vi "Temperature controller top level_v3.vi"() -> ()   [LabVIEW 2015]
uses:
  heating or cooling.vi
  <vilib>/Utility/file.llb/Write Delimited Spreadsheet (DBL).vi
  Heating or cooling global.vi
  <vilib>/Utility/file.llb/Write Delimited Spreadsheet (string).vi
panel:
  in  "?":bool
  in  "Time step":u32=2000
  in  "Comments":string="DTLquad5_run1"
  in  "TSetpoint":sgl=50.0
  in  "file path (dialog if empty)":path=path "C:/Temperature cycling test data/DTLquad5_run2"
  in  "error in":errorcluster
  out "Tcurrent":dbl(slide)=37.65891647338867 scale=0.0..100.0
  out "Tambient":dbl(slide)=23.492000579833984 scale=0.0..100.0
  out "Tambient":sgl=23.492
  out "Tcurrent":sgl=37.658916
  out "error out":errorcluster {"code" format="%.0x"}
  out "Current iteration":i32
  in  "Number of iterations":i32=5
  in  "Current limit":dbl=10.6 caption="Current"
  in  "Voltage":dbl=15.0 format="%#_13g"
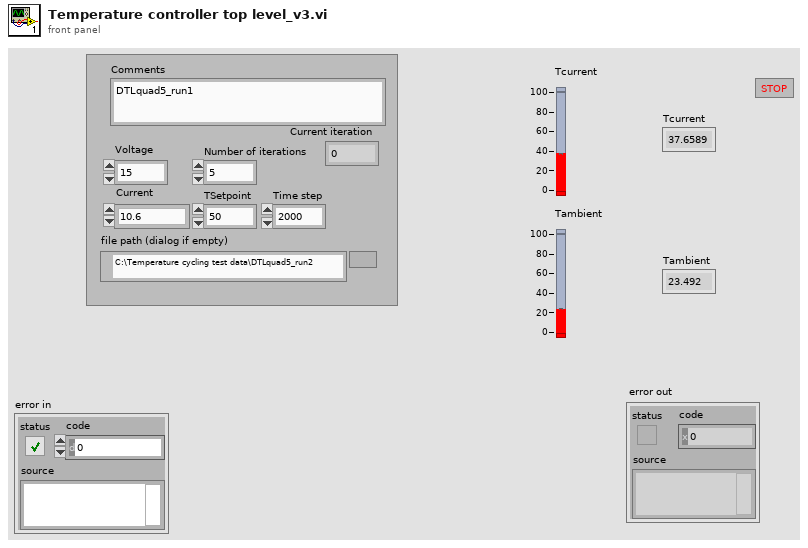
[diagram p1: front panel]
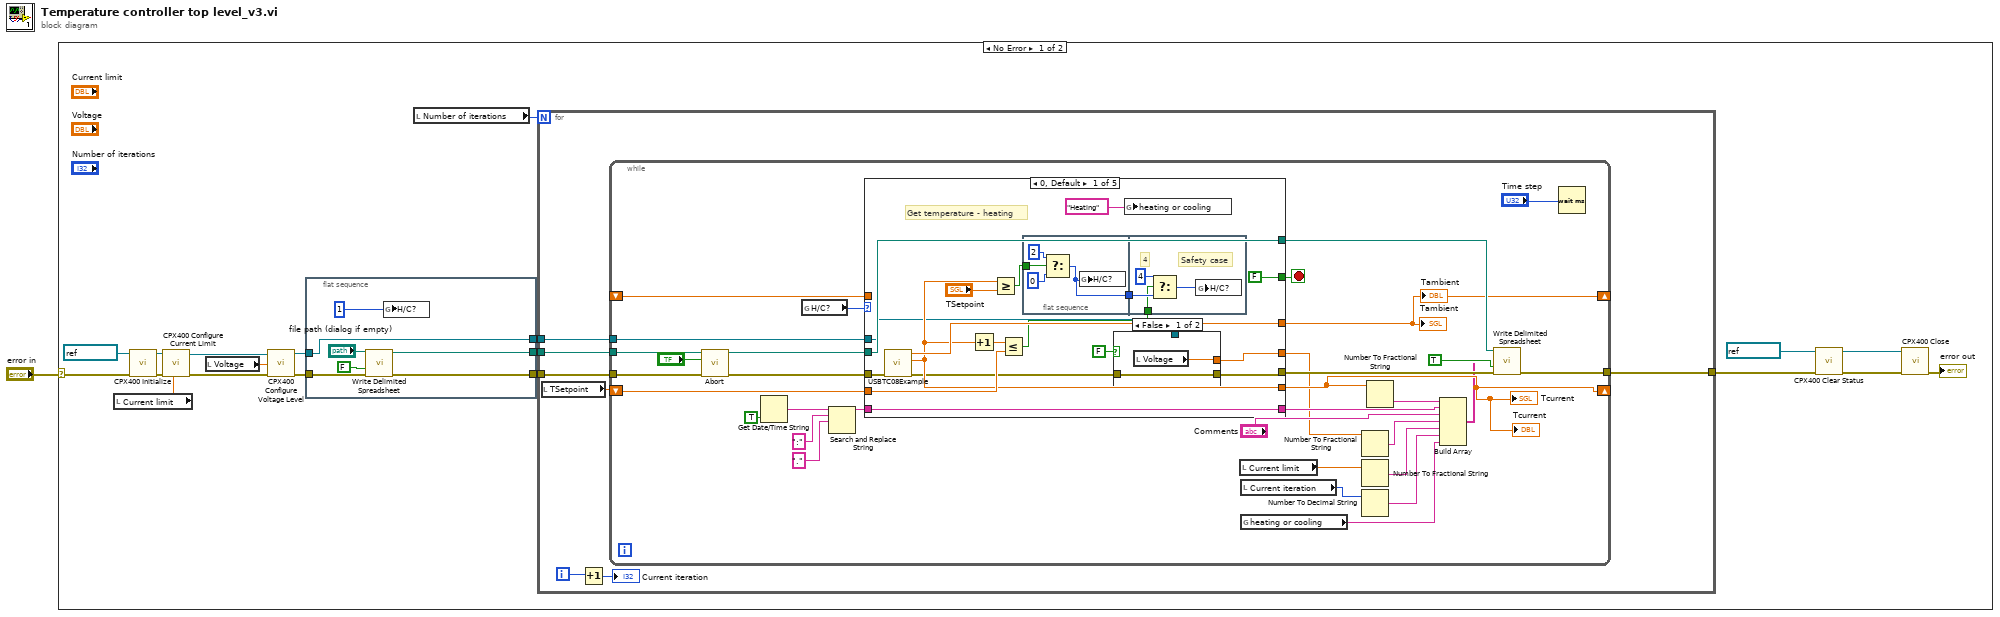
[diagram p0: block diagram]
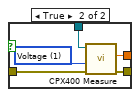
[diagram p2: hidden frame]
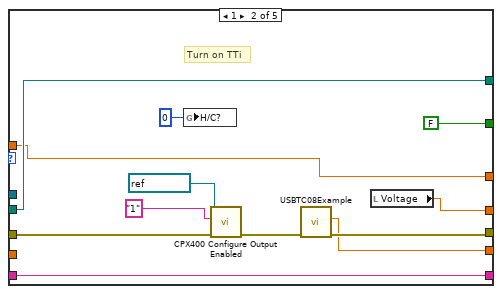
[diagram p3: hidden frame]
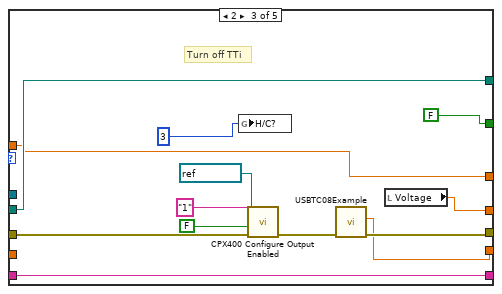
[diagram p4: hidden frame]
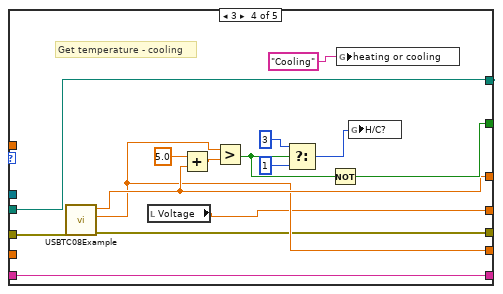
[diagram p5: hidden frame]
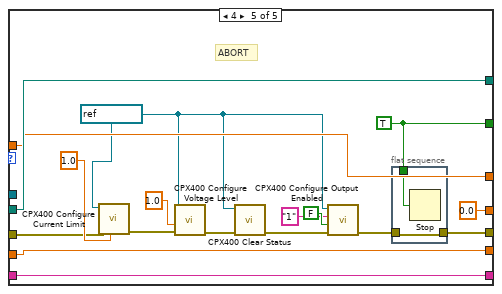
[diagram p6: hidden frame]
diagram:
  n1 = case shown="No Error" "error in" {
    selector: "error in" -> [w7 _]
    frame No Error {
      n2 = local read "Current limit"() -> (w16:dbl)
      n3 = call <instrlib>:"CPX400 Initialize.vi"("error in (no error)"=w7, "resource name"=refnum<k15> "COM5") -> ("error out"=w15:errorcluster, "instrument handle out"=w14:refnum<k15>)  [unwired: 8 in]
      n4 = call <instrlib>:"CPX400 Configure Current Limit.vi"("limit (1.0)"=w16, "error in (no error)"=w15, "instrument handle"=w14) -> ("error out"=w18:errorcluster, "instrument handle out"=w19:refnum<k15>)  [unwired: 7 in]
      n5 = local read "Voltage"() -> (w17:dbl)
      n6 = call <instrlib>:"CPX400 Configure Voltage Level.vi"("error in (no error)"=w18, "level (1.0)"=w17, "instrument handle"=w19) -> ("error out"=w10:errorcluster, "instrument handle out"=w12:refnum<k15>)  [unwired: 7 in]
      n7 = flat-sequence {
        tunnel: w12 -> [w21]
        tunnel: [w24] -> w11
        tunnel: w10 -> [w25]
        tunnel: [w23] -> w9
        tunnel: [w21] -> w6
        frame #0 {
          n8 = call-poly <vilib>:"Write Delimited Spreadsheet.vi"("file path (dialog if empty)"="file path (dialog if empty)", "append to file? (F)"=FALSE, "error in (no error)"=w25) -> ("new file path (Not A Path if cancelled)"=w23:path, "error out"=w24:errorcluster)  [unwired: 11 in]
          n9 = global write "heating or cooling.vi" "H/C?"(u8 1 ("heating or cooling")) -> ()
        }
      }
      n10 = local read "Number of iterations"() -> (w13:i32)
      n11 = for {
        N: w13 -> [_]
        tunnel: w11 -> [w34]
        tunnel: w9 -> [w33]
        tunnel: [w32] -> w5
        tunnel: w6 -> [w28]
        i -> [w30]
        n12 = local read "TSetpoint"() -> (w31:sgl)
        n13 = Increment(x=w30) -> (x+1=→"Current iteration":i32)
        n14 = while {
          tunnel: w34 -> [w37]
          shift-right: [w50] -> _
          shift-left: w31 -> [w65]
          tunnel: w33 -> [w57]
          tunnel: [w56] -> w32
          shift-right: [w53] -> _
          shift-left: _ -> [w54]
          tunnel: w28 -> [w38]
          stop <- w66 stop-if-true
          n15 = call "Abort.vi"("error in"=w37, "stop"="?") -> ("error in 2"=w36:errorcluster)  [unwired: 9 in]
          n16 = Get Date/Time String(want seconds? (F)=TRUE) -> (time string=w63:string)  [unwired: 2 in, 1 out]
          n17 = global read "heating or cooling.vi" "H/C?"() -> (w52:u8)
          n18 = Search and Replace String(input string=w63, search string=":", replace string="." ("replace string (\"\")")) -> (result string=w60:string)  [unwired: 5 in, 3 out]
          n19 = case shown="0, Default" w52 {
            tunnel: w36 -> [w77 w111 w123 w131 w147]
            tunnel: [w73 w101 w113 w128 w151] -> w50
            tunnel: [FALSE ("y") FALSE FALSE w134 w149] -> w66
            tunnel: w65 -> [w83 _ _ _ w151]
            tunnel: w60 -> [w82 w108 w120 w133 w150]
            tunnel: [w82 w108 w120 w133 w150] -> w51
            tunnel: [w81 w107 w119 w132 w153] -> w58
            tunnel: w57 -> [w81 w107 w119 w132 w153]
            tunnel: [w70 w102 w114 w126 w148] -> w55
            tunnel: [w78 w105 w117 w130 w152] -> w53
            tunnel: w54 -> [_ w105 w117 _ w152]
            tunnel: [w69 w100 w112 w125 0.0 ("Voltage")] -> w39
            tunnel: w38 -> [w68 _ _ _ _]
            frame 0, Default {
              # "Get temperature - heating"
              n20 = call "USBTC08Example.vi"("error in"=w77) -> ("error out"=w71:errorcluster, "Tcurrent"=w73:sgl, "Tambient"=w78:sgl)  [unwired: 8 in]
              n21 = Increment(x=w73) -> (x+1=w74:sgl)
              n22 = Greater Or Equal?(x=w73, y="TSetpoint") -> (x >= y?=w79:bool)
              n23 = Less Or Equal?(x=w74, y=w83) -> (x <= y?=w75:bool)
              n24 = flat-sequence {
                tunnel: w79 -> [w93]
                tunnel: [w92] -> w76
                tunnel: w76 -> [w97]
                tunnel: w75 -> [w96]
                frame #0 {
                  n25 = Select(t=2, s=w93, f=0) -> (s? t:f=w92:i32)
                  n26 = global write "heating or cooling.vi" "H/C?"(w92) -> ()
                }
                frame #1 {
                  # "Safety case"
                  # "4"
                  n27 = Select(t=4, s=w96, f=w97) -> (s? t:f=w99:i32)
                  n28 = global write "heating or cooling.vi" "H/C?"(w99) -> ()
                }
              }
              n29 = case shown="False" FALSE {
                tunnel: w71 -> [w86 w91]
                tunnel: [w86 w90] -> w70
                tunnel: [w85 w89] -> w69
                tunnel: w68 -> [_ w87]
                frame False {
                  n30 = local read "Voltage"() -> (w85:dbl)
                }
                frame True {
                  w88 = 1 items=["Voltage"=1, "Current"=0] ("measurement type (Voltage)")
                  n31 = call <instrlib>:"CPX400 Measure.vi"("error in (no error)"=w91, "measurement type (Voltage)"=w88, "instrument handle"=w87) -> ("error out"=w90:errorcluster, "measurement"=w89:dbl)  [unwired: 6 in, 1 out]
                }
              }
              n32 = global write "Heating or cooling global.vi" "heating or cooling"("Heating") -> ()
            }
            frame 1 {
              # "Turn on TTi"
              n33 = global write "heating or cooling.vi" "H/C?"(0) -> ()
              n34 = call <instrlib>:"CPX400 Configure Output Enabled.vi"("error in (no error)"=w111, "channel name (\"1\")"="1" ("channel name (\"1\")"), "instrument handle"=refnum<k15> "COM5" ("resource name")) -> ("error out"=w103:errorcluster)  [unwired: 7 in, 1 out]
              n35 = call "USBTC08Example.vi"("error in"=w103) -> ("error out"=w102:errorcluster, "Tcurrent"=w101:sgl)  [unwired: 8 in, 1 out]
              n36 = local read "Voltage"() -> (w100:dbl)
            }
            frame 2 {
              # "Turn off TTi"
              n37 = global write "heating or cooling.vi" "H/C?"(u8 3 ("heating or cooling")) -> ()
              n38 = call <instrlib>:"CPX400 Configure Output Enabled.vi"("error in (no error)"=w123, "enabled (True)"=FALSE, "channel name (\"1\")"="1" ("channel name (\"1\")"), "instrument handle"=refnum<k15> "COM5" ("resource name")) -> ("error out"=w115:errorcluster)  [unwired: 6 in, 1 out]
              n39 = call "USBTC08Example.vi"("error in"=w115) -> ("error out"=w114:errorcluster, "Tcurrent"=w113:sgl)  [unwired: 8 in, 1 out]
              n40 = local read "Voltage"() -> (w112:dbl)
            }
            frame 3 {
              # "Get temperature - cooling"
              n41 = call "USBTC08Example.vi"("error in"=w131) -> ("error out"=w126:errorcluster, "Tcurrent"=w128:sgl, "Tambient"=w130:sgl)  [unwired: 8 in]
              n42 = local read "Voltage"() -> (w125:dbl)
              n43 = Add(x=sgl 5.0 ("y"), y=w130) -> (x+y=w139:sgl)
              n44 = Greater?(x=w128, y=w139) -> (0:w135:bool)
              n45 = Select(t=u8 3, s=w135, f=u8 1) -> (s? t:f=w129:u8)
              n46 = Not(x=w135) -> (.not. x?=w134:bool)
              n47 = global write "Heating or cooling global.vi" "heating or cooling"("Cooling") -> ()
              n48 = global write "heating or cooling.vi" "H/C?"(w129) -> ()
            }
            frame 4 {
              w149 = TRUE ("y")
              w142 = refnum<k15> "COM5" ("resource name")
              # "ABORT"
              n49 = call <instrlib>:"CPX400 Configure Current Limit.vi"("limit (1.0)"=1.0, "error in (no error)"=w147, "instrument handle"=w142) -> ("error out"=w154:errorcluster)  [unwired: 7 in, 1 out]
              n50 = call <instrlib>:"CPX400 Configure Voltage Level.vi"("error in (no error)"=w154, "level (1.0)"=1.0, "instrument handle"=w142) -> ("error out"=w141:errorcluster)  [unwired: 7 in, 1 out]
              n51 = call <instrlib>:"CPX400 Clear Status.vi"("error in (no error)"=w141, "instrument handle"=w142) -> ("error out"=w140:errorcluster)  [unwired: 8 in, 1 out]
              n52 = call <instrlib>:"CPX400 Configure Output Enabled.vi"("error in (no error)"=w140, "enabled (True)"=FALSE, "channel name (\"1\")"="1" ("channel name (\"1\")"), "instrument handle"=w142) -> ("error out"=w145:errorcluster)  [unwired: 6 in, 1 out]
              n53 = flat-sequence {
                tunnel: w149 -> [w158]
                tunnel: [w157] -> w148
                tunnel: w145 -> [w157]
                frame #0 {
                  n54 = Stop(stop? (T)=w158) -> ()
                }
              }
            }
          }
          "Tcurrent" <- w50
          "Tambient" <- w53
          "Tambient" <- w53
          "Tcurrent" <- w50
          n55 = local read "Current limit"() -> (w46:dbl)
          n56 = local read "Current iteration"() -> (w43:i32)
          n57 = global read "Heating or cooling global.vi" "heating or cooling"() -> (w41:string)
          n58 = Number To Fractional String(number=w39) -> (F-format string=w44:string)  [unwired: 3 in]
          n59 = Number To Fractional String(number=w46) -> (F-format string=w45:string)  [unwired: 3 in]
          n60 = Number To Decimal String(number=w43) -> (decimal integer string=w42:string)  [unwired: 1 in]
          n61 = Number To Fractional String(number=w50) -> (F-format string=w49:string)  [unwired: 3 in]
          n62 = Build Array(w49, w51, "Comments", w44, w45, w42, w41) -> (w47:string[])
          n63 = call-poly <vilib>:"Write Delimited Spreadsheet.vi"("file path (dialog if empty)"=w58, "1D data"=w47, "append to file? (F)"=TRUE, "error in (no error)"=w55) -> ("error out"=w56:errorcluster)  [unwired: 10 in, 1 out]
          n64 = Wait (ms)(milliseconds to wait="Time step") -> ()  [unwired: 1 out]
        }
      }
      n65 = call <instrlib>:"CPX400 Clear Status.vi"("error in (no error)"=w5, "instrument handle"=refnum<k15> "COM5" ("resource name")) -> ("error out"=w4:errorcluster, "instrument handle out"=w2:refnum<k15>)  [unwired: 8 in]
      n66 = call <instrlib>:"CPX400 Close.vi"("error in (no error)"=w4, "instrument handle"=w2) -> ("error out"=→"error out":errorcluster)  [unwired: 9 in]
    }
    frame Error {
    }
  }
